vi "Set Report Header Text.vi"(0 "report in":refnum<class "NI_Standard Report.lvclass">, 5 "left header text":string, 7 "center header text":string, 9 "right header text":string, 11 "error in (no error)":errorcluster, 12 "HTML header size":enum16{"H1", "H2", "H3", "H4", "H5", "H6", "H7"}(ring)=enum."H3", 13 "header placement":enum16{"Top of Document", "Append to Body"}(ring)) -> (4 "report out":refnum<class "NI_Standard Report.lvclass">, 15 "error out":errorcluster)   [LabVIEW 2015, in "NI_Standard Report.lvclass"]
doc: "Sets the text of the report header."
uses:
  <vilib>/Utility/NIReport.llb/Standard Report/NI_Standard Report.lvclass
  <vilib>/Utility/NIReport.llb/Standard Report/NI_Standard Report.lvclass/NI_Standard Report.ctl
  <vilib>/Utility/NIReport.llb/NI_ReportGenerationCore.lvlib
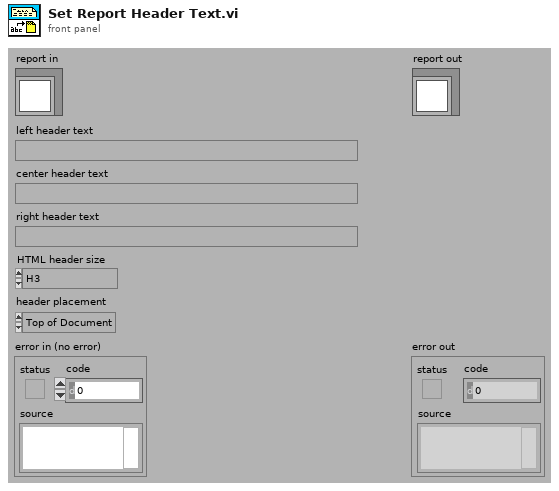
[diagram p1: front panel]
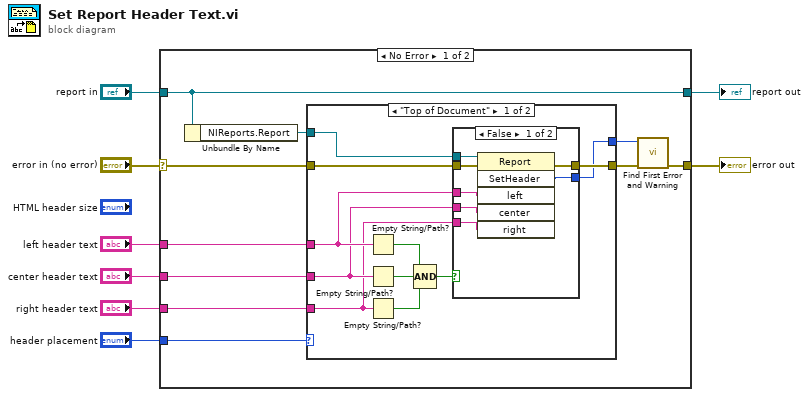
[diagram p0: block diagram]
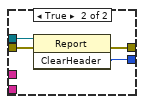
[diagram p2: hidden frame]
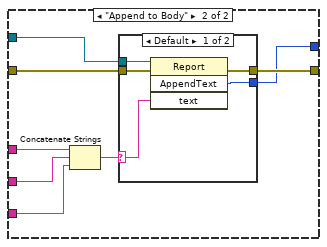
[diagram p3: hidden frame]
diagram:
  n1 = case shown="No Error" "error in (no error)" {
    selector: "error in (no error)" -> [w10 w56]
    tunnel: [w9 w56] -> w7
    tunnel: [w15 w55] -> w5
    tunnel: "report in" -> [w15 w55]
    tunnel: "left header text" -> [w14 _]
    tunnel: "center header text" -> [w13 _]
    tunnel: "right header text" -> [w12 _]
    tunnel: "header placement" -> [w11 _]
    frame No Error {
      n2 = Unbundle By Name(w15) -> ("NIReports.Report"=w16:refnum<k7>)
      n3 = case shown="\"Top of Document\"" w11 {
        tunnel: w14 -> [w25 w44]
        tunnel: w13 -> [w24 w43]
        tunnel: w12 -> [w23 w42]
        tunnel: w10 -> [w22 w48]
        tunnel: [w21 w47] -> w17
        tunnel: [w20 w46] -> w18
        tunnel: w16 -> [w19 w45]
        frame "Top of Document" {
          n4 = Empty String/Path?(string/path=w25) -> (empty?=w28:bool)
          n5 = Empty String/Path?(string/path=w24) -> (empty?=w27:bool)
          n6 = Empty String/Path?(string/path=w23) -> (empty?=w26:bool)
          n7 = Compound Arithmetic op=AND(w28, w27, w26) -> (w29:bool)
          n8 = case shown="False" w29 {
            tunnel: w25 -> [w36 _]
            tunnel: w24 -> [w35 _]
            tunnel: w23 -> [w34 _]
            tunnel: [w33 w37] -> w20
            tunnel: [w32 w38] -> w21
            tunnel: w22 -> [w31 w39]
            tunnel: w19 -> [w30 w40]
            frame False {
              n9 = invoke class="Report" method="SetHeader"(reference=w30, error in=w31, "left"=w36, "center"=w35, "right"=w34) -> (error out=w32:errorcluster, "SetHeader"=w33:i32)  [unwired: 1 in, 4 out]
            }
            frame True {
              n10 = invoke class="Report" method="ClearHeader"(reference=w40, error in=w39) -> (error out=w38:errorcluster, "ClearHeader"=w37:i32)  [unwired: 1 in, 1 out]
            }
          }
        }
        frame "Append to Body" {
          n11 = Concatenate Strings(w44, w43, w42) -> (w41:string)
          n12 = case shown="Default" w41 {
            selector: w41 -> [w49 _]
            tunnel: [w53 _] -> w46
            tunnel: [w52 w54] -> w47
            tunnel: w48 -> [w51 w54]
            tunnel: w45 -> [w50 _]
            frame Default {
              n13 = invoke class="Report" method="AppendText"(reference=w50, error in=w51, "text"=w49) -> (error out=w52:errorcluster, "AppendText"=w53:i32)  [unwired: 1 in, 2 out]
            }
            frame "" {
            }
          }
        }
      }
      n14 = call <vilib>:"Find First Error and Warning.vi"("error in (no error)"=w17, "error code"=w18) -> ("error out"=w9:errorcluster)  [unwired: 1 in, 4 out]
    }
    frame Error {
    }
  }
  "error out" <- w7
  "report out" <- w5
